vi "Task Type.vi"(11 "LoggingManager in":refnum<class "LoggingManager.lvclass">) -> (2 "Task Type":string)   [LabVIEW 2020, in "VolatusDataLogger.lvlib" / "LoggingManager.lvclass"]
uses:
  LoggingManager.lvclass
  LoggingManager.lvclass/LoggingManager.ctl
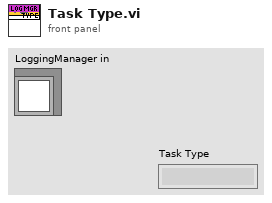
[diagram p1: front panel]
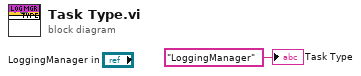
[diagram p0: block diagram]
diagram:
  "Task Type" <- "LoggingManager" ("Task Type")
